vi "Listbox-Click to add.vi"(0 "ListBox":refnum<vi>, 5 "Strings":string[](array[string]), 9 "Prompt":string="Click to add", 11 "Row":i32) -> (4 "reference out":refnum<vi>)   [LabVIEW 2020]
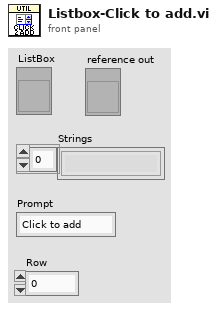
[diagram p1: front panel]
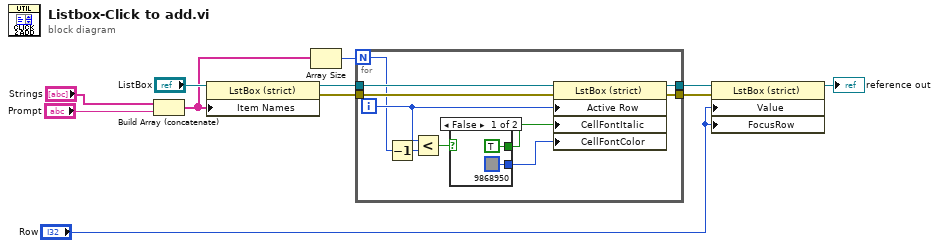
[diagram p0: block diagram]
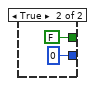
[diagram p2: hidden frame]
diagram:
  n1 = Build Array (concatenate)("Strings", "Prompt") -> (w7:string[])
  n2 = property on="Property Node" class="LstBox (strict)"(reference="ListBox", "Item Names"=w7) -> (reference out=w6:refnum<vi>, error out=w5:errorcluster)  [unwired: 1 in]
  n3 = Array Size(array=w7) -> (size(s)=w8:i32)
  n4 = for {
    N: w8 -> [w14]
    tunnel: w6 -> [w21]
    tunnel: w5 -> [w18]
    tunnel: [w13] -> w4
    tunnel: [w12] -> w3
    i -> [w16]
    n5 = Decrement(x=w14) -> (x-1=w15:i32)
    n6 = Less?(x=w16, y=w15) -> (x < y?=w17:bool)
    n7 = case shown="False" w17 {
      tunnel: [TRUE FALSE] -> w20
      tunnel: [u32 9868950 u32 0] -> w19
      frame False {
      }
      frame True {
      }
    }
    n8 = property on="Property Node" class="LstBox (strict)"(reference=w21, error in=w18, "Active Row"=w16, "CellFontItalic"=w20, "CellFontColor"=w19) -> (reference out=w13:refnum<vi>, error out=w12:errorcluster)
  }
  n9 = property on="Property Node" class="LstBox (strict)"(reference=w4, error in=w3, "Value"="Row", "FocusRow"="Row") -> (reference out=→"reference out":refnum<vi>)  [unwired: 1 out]
